vi "READ FILE TEST.vi"() -> ()   [LabVIEW 2020]
uses:
  F:/MY FILE/FaceRecognitionDotNet 1.2.3.10/FaceRecognitionDotNet/FaceRecognition Class/dll/FaceRecognitionDotNet.dll
  FaceRecognitionDotNet/FaceRecognition Class/dll/FaceRecognitionDotNet.dll
  FaceRecognitionDotNet/FaceRecognition Class/ctl/LocationModel.ctl
  FaceRecognitionDotNet/FaceRecognition Class/FaceRecognition.lvclass
panel:
  in  "mode path":path=path "F:/MY FILE/FaceRecognitionDotNet 1.2.3.10/FaceRecognitionDotNet/models"
  out "ms 5":u32
  out "ms 4":u32
  out "ms 3":u32
  out "ms":u32
  in  "numberOfTimesToUpsample":i32
  out "CompareFace":bool
  out "FaceDistance":dbl
  out "CompareFaces":bool[](array[boolean])
  out "CurrentArray":dbl[](array[numeric])
  in  "LoadEncoding":bool
  in  "Encoding":bool
  in  "Landmark":bool
  in  "Open Button":bool
  in  "Cancel Button":bool
  in  "IMAGE Path":path
  out "Image":T1(plugin-control)
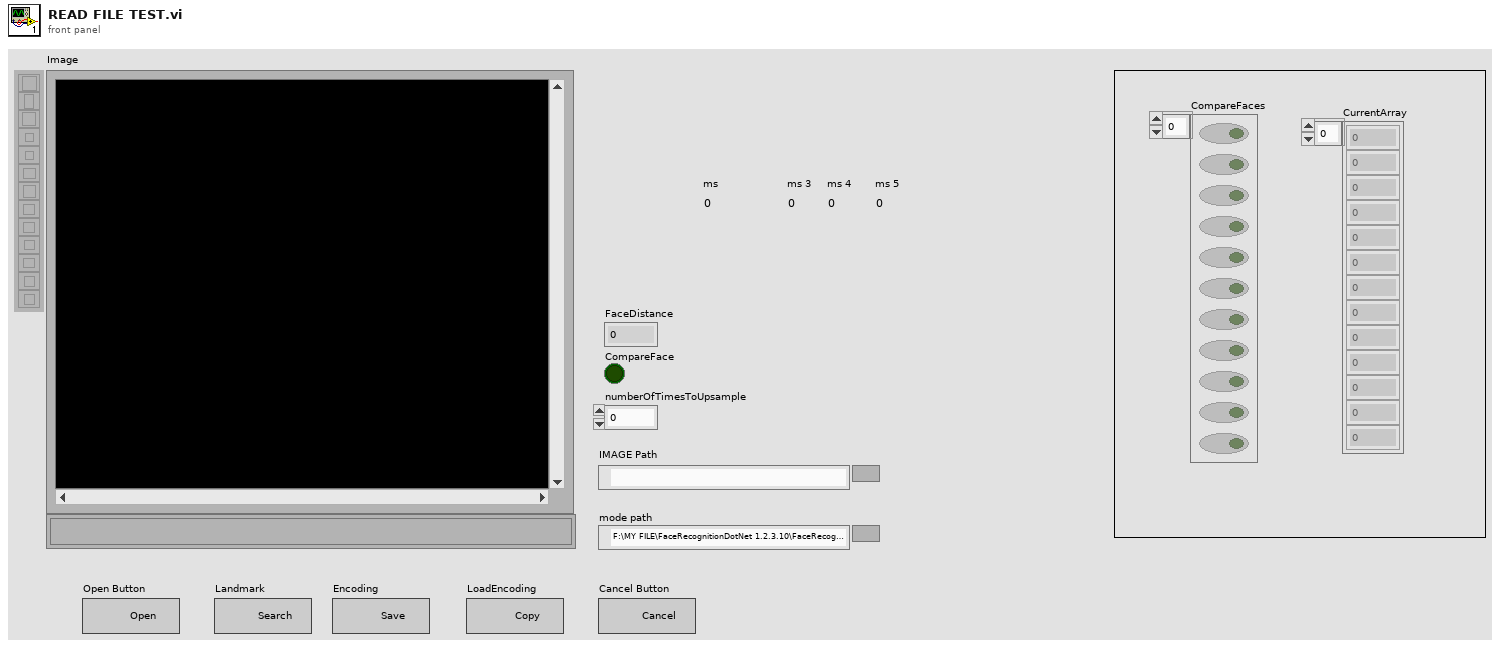
[diagram p1: front panel]
types:
  T1 = typedef "IMAQ Image.ctl" = refnum<image>
  T2 = typedef "Image Type" = u32
  T3 = cluster{"Desired Font (Application)":enum16{"User-specified Font", "Application Font", "System Font", "Dialog Font"}, "[User-specified Font]":cluster{"Font Name":string, "Size":i16, "Strikeout?":bool, "Italic?":bool, "Underline?":bool, "Outline?":bool, "Shadow?":bool, "Bold?":bool, "Rotation Angle":dbl}, "Horizontal Alignment":i16, "Vertical Alignment":i16}
  T4 = typedef "FaceRecognitionDotNet.lvlib/FaceRecognition.lvclass/LocationModel.ctl" = i32
  T5 = cluster{"Left":i32, "Top":i32, "Right":i32, "Bottom":i32}
  T6 = typedef "FaceRecognitionDotNet.lvlib/FaceRecognition.lvclass/FacePart.ctl" = i32
  T7 = typedef "FaceRecognitionDotNet.lvlib/FaceRecognition.lvclass/Point.ctl" = cluster{"X":sgl, "Y":sgl}
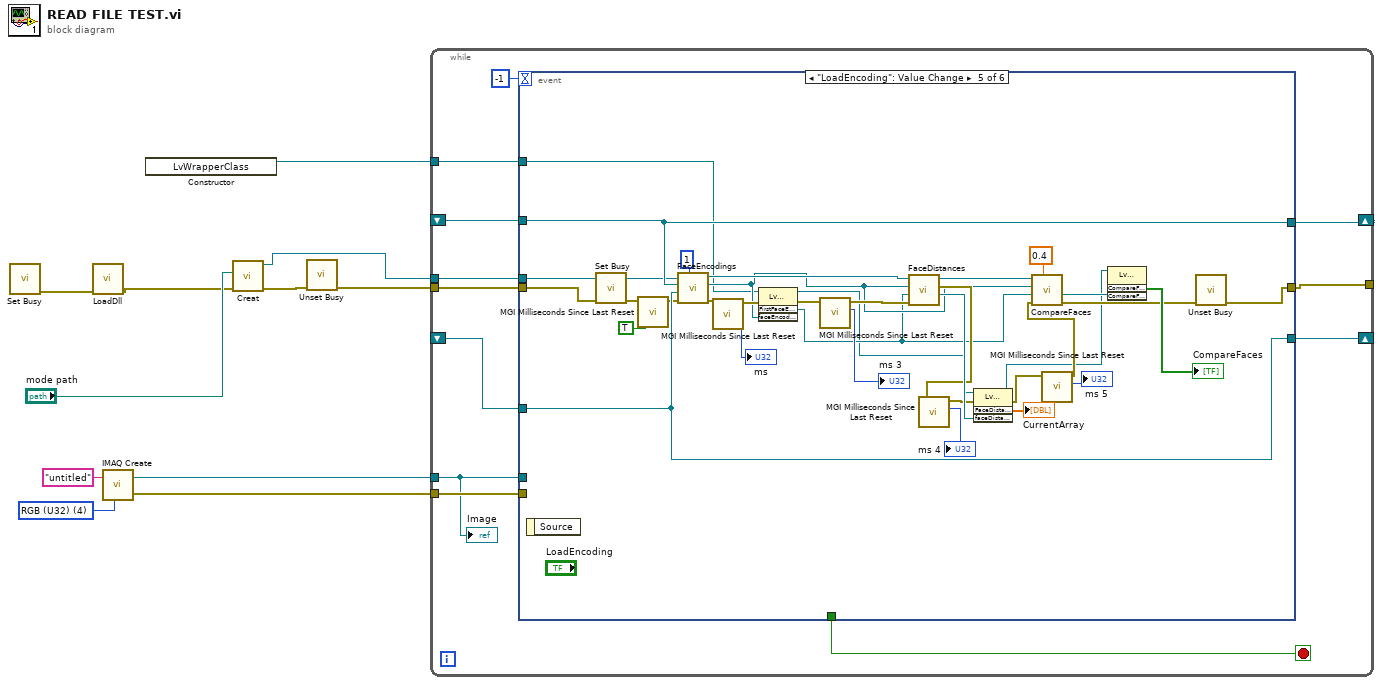
[diagram p0: block diagram]
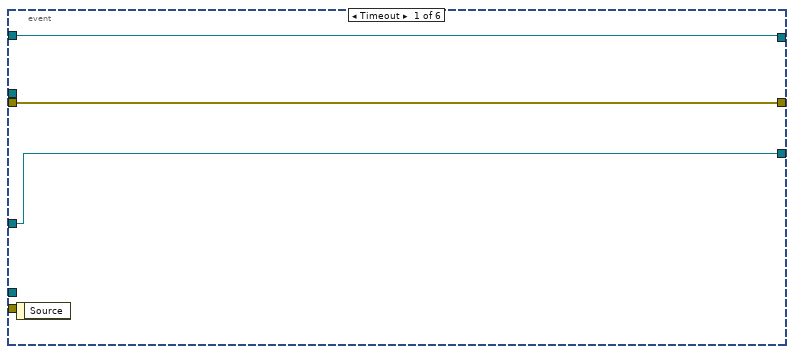
[diagram p2: hidden frame]
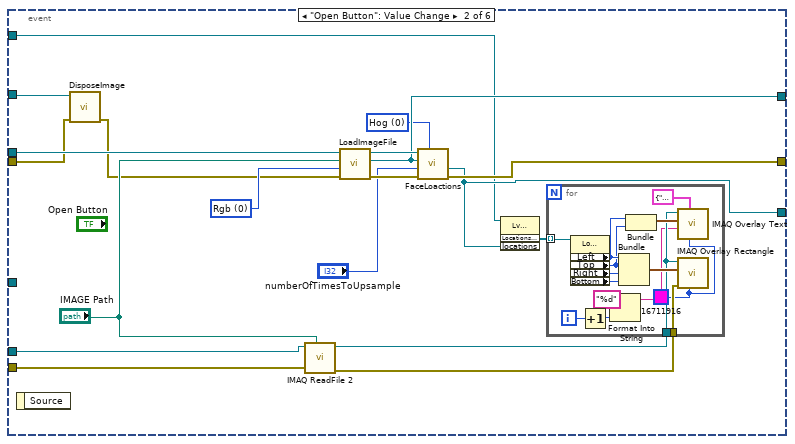
[diagram p3: hidden frame]
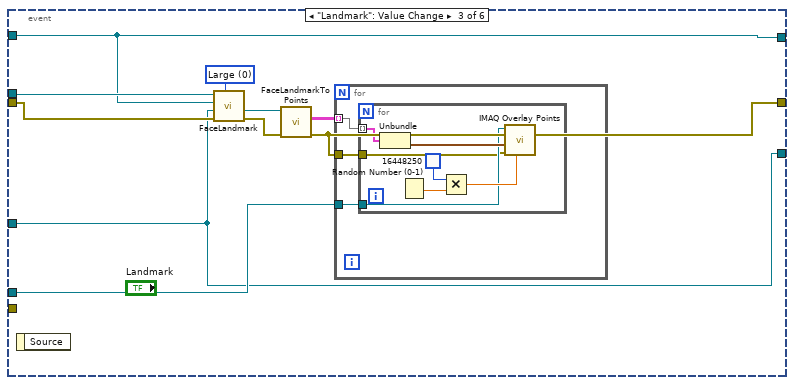
[diagram p4: hidden frame]
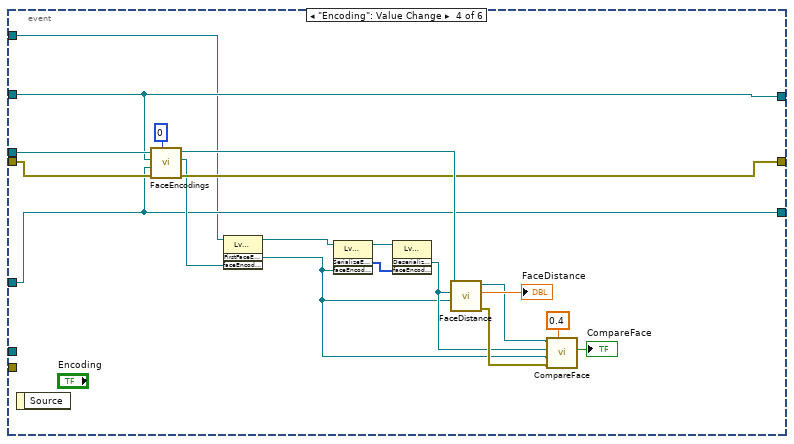
[diagram p5: hidden frame]
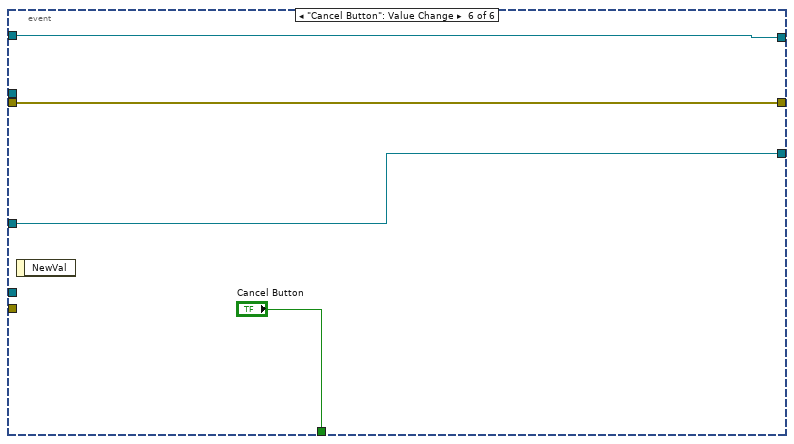
[diagram p6: hidden frame]
diagram:
  w8 = T2 4 items=["Grayscale (U8)", "Grayscale (I16)", "Grayscale (SGL)", "Complex (CSG)", "RGB (U32)", "HSL (U32)", "RGB (U64)", "Grayscale (U16)"] ("Image Type")
  n1 = call <vilib>:"Set Busy.vi"() -> ("error out"=w4:errorcluster)  [unwired: 10 in, 1 out]
  n2 = call "LoadDll.vi"("error in (no error)"=w4) -> ("error out"=w3:errorcluster)  [unwired: 10 in]
  n3 = call "IMAQ Create"("Image Name"="untitled", "Image Type"=w8) -> ("New Image"=w11:T1, "error out"=w10:errorcluster)  [unwired: 3 in]
  n4 = constructor class="LvWrapperClass"() -> (reference out=w1:refnum<k24>)  [unwired: 3 in, 2 out]
  n5 = call "Creat.vi"("error in (no error)"=w3, "mode path"="mode path") -> ("error out"=w6:errorcluster, "FaceRecognition out"=w7:refnum<class "FaceRecognition.lvclass">)  [unwired: 8 in]
  n6 = call <vilib>:"Unset Busy.vi"("error in (no error)"=w6) -> ("error out"=w2:errorcluster)  [unwired: 10 in]
  n7 = while {
    tunnel: w7 -> [w22]
    tunnel: w2 -> [w21]
    tunnel: w11 -> [w19]
    tunnel: w10 -> [w20]
    tunnel: [w18] -> _
    shift-right: [w16] -> _
    shift-left: _ -> [w15]
    shift-right: [w14] -> _
    shift-left: _ -> [w13]
    tunnel: w1 -> [w12]
    stop <- w23 stop-if-true
    n8 = event shown="[4] \"LoadEncoding\": Value Change" {
      selector: _ -> [_ _ _ _ _ _]
      dyn-events: _ -> [_ _ _ _ _ _]
      timeout: -1 -> [_ _ _ _ _ _]
      tunnel: [_ _ _ _ _ "Cancel Button"] -> w23
      tunnel: w22 -> [_ w45 w70 w99 w130 _]
      tunnel: w21 -> [w24 w37 w69 w97 w121 w136]
      tunnel: w19 -> [_ w44 w64 _ _ _]
      tunnel: w20 -> [_ w43 _ _ _ _]
      tunnel: [w24 w33 w63 w93 w123 w136] -> w18
      tunnel: [w26 w35 w68 w96 w133 w135] -> w16
      tunnel: w15 -> [w26 w38 w68 w96 w133 w135]
      tunnel: [w25 w29 w61 w85 w122 w134] -> w14
      tunnel: w13 -> [w25 _ w61 w85 w122 w134]
      tunnel: w12 -> [_ w27 _ w81 w100 _]
      event Timeout {
        n9 = event-data() -> ()  [unwired: 1 in, 1 out]
      }
      event "Open Button": Value Change {
        w34 = T4 0 items=["Hog", "Cnn"] ("model")
        w42 = 0 items=["Rgb", "Greyscale"] ("mode")
        n10 = event-data() -> ()  [unwired: 1 in, 1 out]
        n11 = call "DisposeImage.vi"("error in (no error)"=w37, "Image in"=w38) -> ("error out"=w36:errorcluster)  [unwired: 9 in]
        n12 = call "IMAQ ReadFile 2"("File Path"="IMAGE Path", "error in (no error)"=w43, "Image"=w44) -> ("error out"=w32:errorcluster, "Image Out"=w31:T1)  [unwired: 4 in, 3 out]
        n13 = call "LoadImageFile.vi"("error in (no error)"=w36, "mode"=w42, "FilePath"="IMAGE Path", "FaceRecognition in"=w45) -> ("error out"=w39:errorcluster, "LoadImageFile"=w35:refnum<k24>, "FaceRecognition out"=w40:refnum<class "FaceRecognition.lvclass">)  [unwired: 5 in]
        n14 = call "FaceLoactions.vi"("model"=w34, "error in (no error)"=w39, "numberOfTimesToUpsample"="numberOfTimesToUpsample", "image"=w35, "FaceRecognition in"=w40) -> ("error out"=w33:errorcluster, "FaceLocations"=w29:refnum<k24>)  [unwired: 3 in, 2 out]
        n15 = invoke class="LvWrapperClass" method="LocationsArray"(reference=w27, "locations"=w29) -> ("LocationsArray"=w28:refnum<k24>[])  [unwired: 2 in, 3 out]
        n16 = for {
          tunnel: w32 -> [w60]
          tunnel: w31 -> [w52]
          tunnel: w28 -> [w59] mode=indexing
          i -> [w51]
          w47 = u32 16711916 ("Color")
          n17 = property class="Location"(reference=w59) -> ("Left"=w55:i32, "Top"=w54:i32, "Right"=w57:i32, "Bottom"=w58:i32)  [unwired: 1 in, 2 out]
          n18 = Increment(x=w51) -> (x+1=w50:i32)
          n19 = Format Into String(format string="%d", w50) -> (resulting string=w48:string)  [unwired: 2 in, 1 out]
          n20 = Bundle("Left"=w55, "Top"=w54, "Right"=w57, "Bottom"=w58) -> (w56:T5)  [unwired: 1 in]
          n21 = Bundle("Left"=w55, "Top"=w54) -> (w53:cluster{"Left":i32, "Top":i32})  [unwired: 1 in]
          n22 = call "IMAQ Overlay Text"("Text Color (black)"=w47, "Font, Size & Style"=T3 {"Desired Font (Application)"=enum."System Font", "[User-specified Font]"={"Font Name"="Tahoma", "Size"=100, "Strikeout?"=FALSE, "Italic?"=FALSE, "Underline?"=FALSE, "Outline?"=FALSE, "Shadow?"=FALSE, "Bold?"=FALSE, "Rotation Angle"=0.0}, "Horizontal Alignment"=0, "Vertical Alignment"=0}, "String"=w48, "Origin"=w53, "Image"=w52) -> ()  [unwired: 5 in, 2 out]
          n23 = call "IMAQ Overlay Rectangle"("Color"=w47, "error in (no error)"=w60, "Rectangle"=w56, "Image"=w52) -> ()  [unwired: 6 in, 2 out]
        }
      }
      event "Landmark": Value Change {
        w67 = 0 items=["Large", "Small"] ("model")
        n24 = event-data() -> ()  [unwired: 1 in, 1 out]
        n25 = call "FaceLandmark.vi"("model"=w67, "error in (no error)"=w69, "FaceLocations"=w61, "FaceImage"=w68, "FaceRecognition in"=w70) -> ("error out"=w66:errorcluster, "FaceLandmark"=w62:refnum<k24>)  [unwired: 3 in, 2 out]
        n26 = call "FaceLandmarkToPoints.vi"("error in (no error)"=w66, "FaceLandmark"=w62) -> ("error out"=w63:errorcluster, "FaceLandmarkArray"=w65:cluster{"item":T6, T7[]}[][])  [unwired: 8 in]
        n27 = for {
          tunnel: w65 -> [w73] mode=indexing
          tunnel: w64 -> [w72]
          tunnel: w63 -> [w71]
          n28 = for {
            tunnel: w73 -> [w80] mode=indexing
            tunnel: w72 -> [w75]
            tunnel: w71 -> [w74]
            n29 = Unbundle(w80) -> (w79:T7[])  [unwired: 1 out]
            n30 = Random Number (0-1)() -> (number: 0 to 1=w78:dbl)
            n31 = Multiply(x=u32 16448250, y=w78) -> (x*y=w76:dbl)
            n32 = call "IMAQ Overlay Points"("Color"=w76, "error in (no error)"=w74, "Array of Points"=w79, "Image"=w75) -> ()  [unwired: 6 in, 2 out]
          }
        }
      }
      event "Encoding": Value Change {
        n33 = event-data() -> ()  [unwired: 1 in, 1 out]
        n34 = call "FaceEncodings.vi"("numJitters"=0, "error in (no error)"=w97, "knownFaceLocation"=w85, "image"=w96, "FaceRecognition in"=w99) -> ("error out"=w93:errorcluster, "FaceEncodings"=w89:refnum<k24>, "FaceRecognition out"=w95:refnum<class "FaceRecognition.lvclass">)  [unwired: 4 in]
        n35 = invoke class="LvWrapperClass" method="FirstFaceEncoding"(reference=w81, "faceEncodings"=w89) -> (reference out=w83:refnum<k24>, "FirstFaceEncoding"=w82:refnum<k24>)  [unwired: 2 in, 2 out]
        n36 = invoke class="LvWrapperClass" method="SerializeEncoding"(reference=w83, "faceEncoding"=w82) -> (reference out=w84:refnum<k24>, "SerializeEncoding"=w92:u8[])  [unwired: 2 in, 2 out]
        n37 = invoke class="LvWrapperClass" method="DeserializeEncoding"(reference=w84, "faceEncoding"=w92) -> ("DeserializeEncoding"=w88:refnum<k24>)  [unwired: 2 in, 3 out]
        n38 = call "FaceDistance.vi"("faceToCompare"=w82, "FaceEncoding"=w88, "FaceRecognition in"=w95) -> ("error out"=w90:errorcluster, "FaceDistance"=→"FaceDistance":dbl, "FaceRecognition out"=w91:refnum<class "FaceRecognition.lvclass">)  [unwired: 6 in]
        n39 = call "CompareFace.vi"("tolerance"=0.4, "error in (no error)"=w90, "faceEncodingToCheck"=w82, "knownFaceEncoding"=w88, "FaceRecognition in"=w91) -> ("CompareFace"=→"CompareFace":bool)  [unwired: 4 in, 2 out]
      }
      event "LoadEncoding": Value Change {
        n40 = event-data() -> ()  [unwired: 1 in, 1 out]
        n41 = call <vilib>:"Set Busy.vi"("error in (no error)"=w121) -> ("error out"=w120:errorcluster)  [unwired: 9 in, 1 out]
        n42 = call <userlib>:"MGI Milliseconds Since Last Reset.vi"("Reset (F)"=TRUE, "Error In"=w120) -> ("Error Out"=w119:errorcluster)  [unwired: 4 in, 1 out]
        n43 = call "FaceEncodings.vi"("numJitters"=1, "error in (no error)"=w119, "knownFaceLocation"=w122, "image"=w133, "FaceRecognition in"=w130) -> ("error out"=w117:errorcluster, "FaceEncodings"=w106:refnum<k24>, "FaceRecognition out"=w132:refnum<class "FaceRecognition.lvclass">)  [unwired: 4 in]
        n44 = call <userlib>:"MGI Milliseconds Since Last Reset.vi"("Error In"=w117) -> ("ms"=→"ms":u32, "Error Out"=w116:errorcluster)  [unwired: 5 in]
        n45 = invoke class="LvWrapperClass" method="FirstFaceEncoding"(reference=w100, error in=w116, "faceEncodings"=w106) -> (reference out=w102:refnum<k24>, error out=w104:errorcluster, "FirstFaceEncoding"=w105:refnum<k24>)  [unwired: 1 in, 1 out]
        n46 = call <userlib>:"MGI Milliseconds Since Last Reset.vi"("Error In"=w104) -> ("ms"=→"ms 3":u32, "Error Out"=w115:errorcluster)  [unwired: 5 in]
        n47 = call "FaceDistances.vi"("error in (no error)"=w115, "faceToCompare"=w105, "faceEncodings"=w106, "FaceRecognition in"=w132) -> ("error out"=w112:errorcluster, "FaceDistances"=w125:refnum<k24>, "FaceRecognition out"=w131:refnum<class "FaceRecognition.lvclass">)  [unwired: 5 in]
        n48 = call <userlib>:"MGI Milliseconds Since Last Reset.vi"("Error In"=w112) -> ("ms"=→"ms 4":u32, "Error Out"=w111:errorcluster)  [unwired: 5 in]
        n49 = invoke class="LvWrapperClass" method="FaceDistanceArray"(reference=w102, error in=w111, "faceDistances"=w125) -> (reference out=w101:refnum<k24>, error out=w109:errorcluster, "FaceDistanceArray"=→"CurrentArray":dbl[])  [unwired: 1 in, 1 out]
        n50 = call <userlib>:"MGI Milliseconds Since Last Reset.vi"("Error In"=w109) -> ("ms"=→"ms 5":u32, "Error Out"=w108:errorcluster)  [unwired: 5 in]
        n51 = call "CompareFaces.vi"("tolerance"=0.4, "error in (no error)"=w108, "faceEncodingToCheck"=w105, "knownFaceEncodings"=w106, "FaceRecognition in"=w131) -> ("error out"=w124:errorcluster, "CompareFaces"=w127:refnum<k24>)  [unwired: 4 in, 1 out]
        n52 = invoke class="LvWrapperClass" method="CompareFaceArray"(reference=w101, "CompareFaces"=w127) -> ("CompareFaceArray"=→"CompareFaces":bool[])  [unwired: 2 in, 3 out]
        n53 = call <vilib>:"Unset Busy.vi"("error in (no error)"=w124) -> ("error out"=w123:errorcluster)  [unwired: 10 in]
      }
      event "Cancel Button": Value Change {
        n54 = event-data() -> ()  [unwired: 1 in, 1 out]
      }
    }
    "Image" <- w19
  }
